vi "plaot slot line.vi"(4 "测试条件out":T3, 6 "粉尘特性":T2, 7 "unit":string, 8 "error in (no error)":errorcluster, 9 "max slop value":cluster{"X":dbl, "Y":dbl}[](array[cluster]), 10 "max slop":dbl, 11 "plot graph":refnum<vi>) -> (0 "error out":errorcluster, 1 "测试条件":string, 2 "intercept":dbl, 3 "dp/dt":string)   [LabVIEW 2011]
panel:
  out "text rect":T1 caption="文本矩形"
  out "rect":T1 caption="矩形"
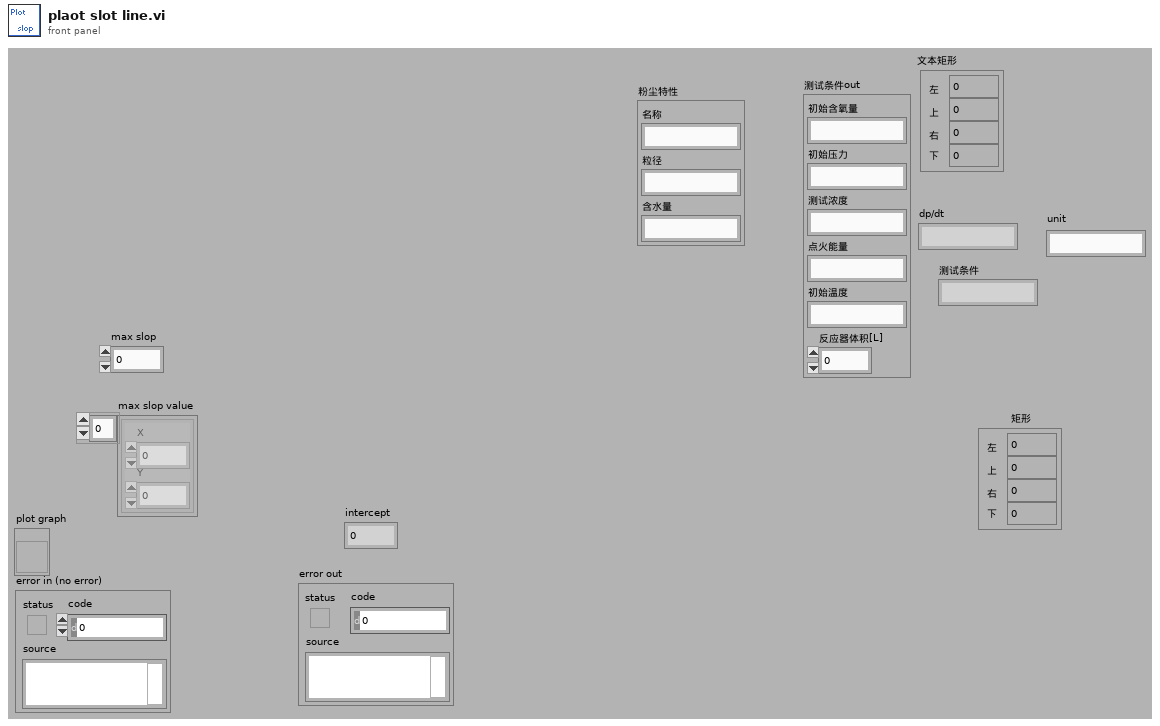
[diagram p1: front panel]
types:
  T1 = cluster{"left":i16, "top":i16, "right":i16, "bottom":i16}
  T2 = typedef "粉尘特性.ctl" = cluster{"名称":string, "粒径":string, "含水量":string}
  T3 = typedef "测试条件.ctl" = cluster{"初始含氧量":string, "初始压力":string, "测试浓度":string, "点火能量":string, "初始温度":string, "反应器体积[L]":dbl}
  T4 = cluster{"horizontal":enum16{"left", "center", "right"}, "vertical":enum16{"top", "center", "bottom"}}
  T5 = enum16{"User-specified Font", "Application Font", "System Font", "Dialog Font"}
  T6 = typedef "LVRectTypeDef.ctl" = cluster{"left":i16, "top":i16, "right":i16, "bottom":i16}
  T7 = typedef "LVPoint32TypeDef.ctl" = cluster{"Horizontal":i32, "Vertical":i32}
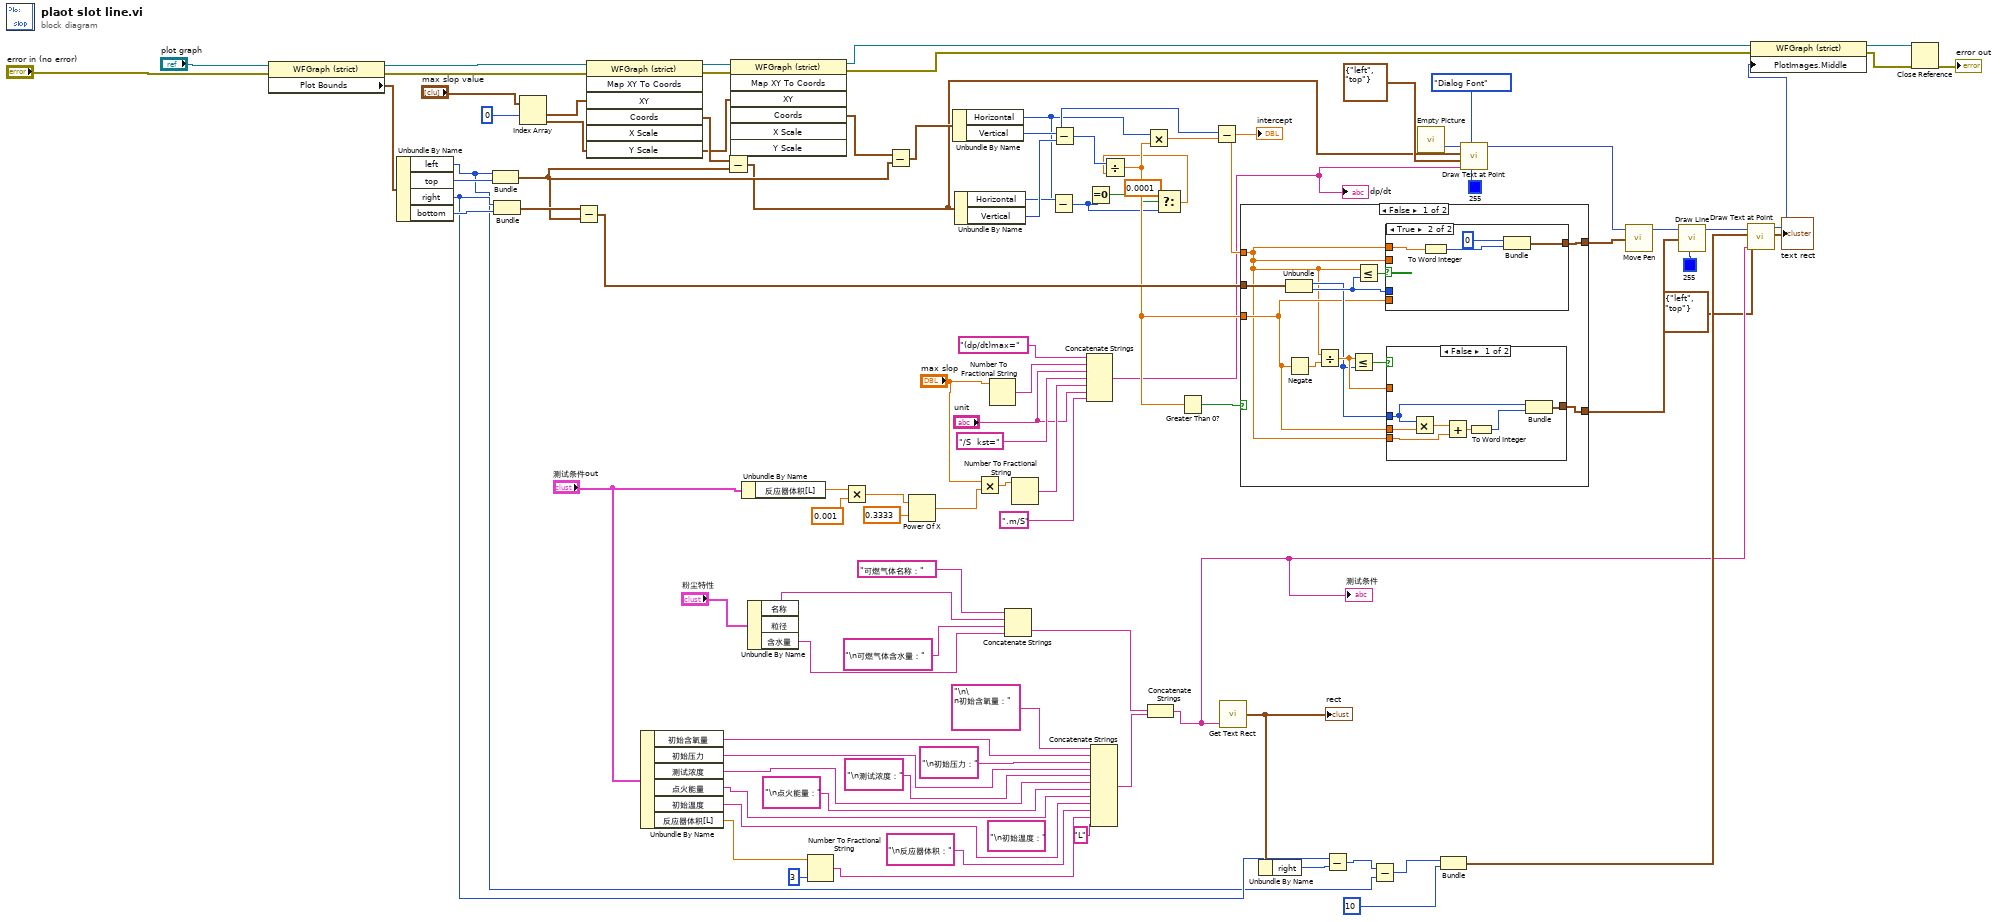
[diagram p0: block diagram]
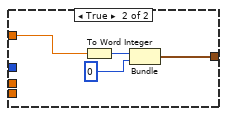
[diagram p2: hidden frame]
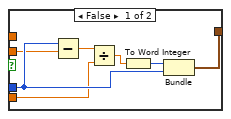
[diagram p3: hidden frame]
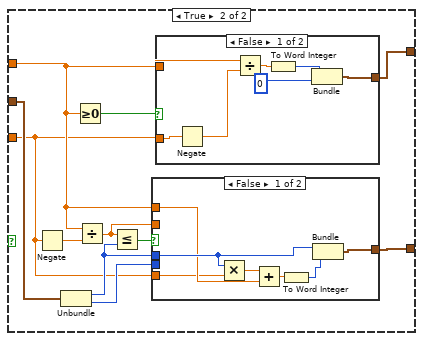
[diagram p4: hidden frame]
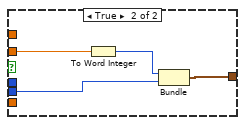
[diagram p5: hidden frame]
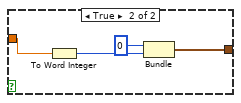
[diagram p6: hidden frame]
diagram:
  (unwired) "\n初始温度：" ("字符串")
  n1 = property class="WFGraph (strict)"(reference="plot graph", error in="error in (no error)") -> (reference out=w89:refnum<vi>, error out=w63:errorcluster, "Plot Bounds"=w88:T6)
  n2 = Unbundle By Name(w88) -> ("left"=w6:i16, "top"=w8:i16, "right"=w10:i16, "bottom"=w83:i16)
  n3 = Bundle("left"=w6, "top"=w8) -> (w81:cluster{"left":i16, "top":i16})  [unwired: 1 out]
  n4 = Bundle("right"=w10, "bottom"=w83) -> (w82:cluster{"right":i16, "bottom":i16})  [unwired: 1 out]
  n5 = Index Array(array="max slop value", index #1=0 ("index")) -> (element #1=w96:cluster{"X":dbl, "Y":dbl}, element #2=w77:cluster{"X":dbl, "Y":dbl})  [unwired: 1 in]
  n6 = Subtract(x=w82, y=w81) -> (x-y=w78:cluster{i16, i16})
  n7 = invoke class="WFGraph (strict)" method="Map XY To Coords"(reference=w89, error in=w63, "XY"=w96) -> (reference out=w92:refnum<vi>, error out=w91:errorcluster, "Coords"=w90:T7)  [unwired: 4 in, 4 out]
  n8 = Unbundle By Name("测试条件out") -> ("初始含氧量"=w30:string, "初始压力"=w27:string, "测试浓度"=w25:string, "点火能量"=w23:string, "初始温度"=w22:string, "反应器体积[L]"=w20:dbl)
  n9 = Subtract(x=w90, y=w81) -> (x-y=w54:T7)
  n10 = invoke class="WFGraph (strict)" method="Map XY To Coords"(reference=w92, error in=w91, "XY"=w77) -> (reference out=w68:refnum<vi>, error out=w62:errorcluster, "Coords"=w87:T7)  [unwired: 4 in, 4 out]
  n11 = Unbundle By Name("测试条件out") -> ("反应器体积[L]"=w40:dbl)
  n12 = Unbundle By Name("粉尘特性") -> ("名称"=w34:string, "含水量"=w31:string)  [unwired: 1 out]
  n13 = Number To Fractional String(number=w20, precision (6)=i16 3 ("精度(6)")) -> (F-format string=w19:string)  [unwired: 2 out]
  n14 = Multiply(x=w40, y=0.001) -> (x*y=w39:dbl)
  n15 = Subtract(x=w87, y=w81) -> (x-y=w71:T7)
  n16 = Power Of X(1:0.3333 ("x"), 2:w39) -> (0:w37:dbl)
  n17 = Unbundle By Name(w71) -> ("Horizontal"=w84:i32, "Vertical"=w86:i32)
  n18 = Unbundle By Name(w54) -> ("Horizontal"=w94:i32, "Vertical"=w95:i32)
  n19 = Multiply(x="max slop", y=w37) -> (x*y=w44:dbl)
  n20 = Number To Fractional String(number="max slop") -> (F-format string=w48:string)  [unwired: 3 out]
  n21 = Concatenate Strings("可燃气体名称：" ("字符串"), w34, "\n可燃气体含水量：" ("字符串"), w31) -> (w18:string)
  n22 = Number To Fractional String(number=w44) -> (F-format string=w45:string)  [unwired: 3 out]
  n23 = Subtract(x=w84, y=w94) -> (x-y=w58:i32)
  n24 = Subtract(x=w86, y=w95) -> (x-y=w93:i32)
  n25 = Concatenate Strings("(dp/dt)max=" ("string"), w48, "unit", "/S  kst=" ("字符串"), w45, "unit", ".m/S" ("字符串")) -> (w69:string)
  "dp/dt" <- w69
  n26 = Equal To 0?(x=w58) -> (x = 0?=w60:bool)
  n27 = Concatenate Strings("\n\n初始含氧量：" ("字符串"), w30, "\n初始压力：" ("字符串"), w27, "\n测试浓度：" ("字符串"), w25, "\n点火能量：" ("字符串"), w23, w22, "\n反应器体积：" ("字符串"), w19, "L" ("字符串")) -> (w17:string)
  n28 = Concatenate Strings(w18, w17) -> (w12:string)
  "测试条件" <- w12
  n29 = Select(t=0.0001, s=w60, f=w58) -> (s? t:f=w57:dbl)
  n30 = Divide(x=w93, y=w57) -> (x/y=w70:dbl)
  n31 = Multiply(x=w84, y=w70) -> (x*y=w85:dbl)
  n32 = Greater Than 0?(x=w70) -> (x > 0?=w80:bool)
  n33 = Subtract(x=w86, y=w85) -> (x-y=w79:dbl)
  "intercept" <- w79
  n34 = call <vilib>:"Get Text Rect.vi"("text"=w12) -> ("rect"=w16:T1)  [unwired: 5 in, 3 out]
  "rect" <- w16
  n35 = case shown="False" w80 {
    tunnel: w79 -> [w99 w131]
    tunnel: w78 -> [w107 w135]
    tunnel: w70 -> [w100 w130]
    tunnel: [w98 w139] -> w74
    tunnel: [w97 w140] -> w76
    frame False {
      n36 = Unbundle(w107) -> (w101:i16, w102:i16)
      n37 = Negate(x=w100) -> (-x=w105:dbl)
      n38 = Divide(x=w99, y=w105) -> (x/y=w103:dbl)
      n39 = Less Or Equal?(x=w103, y=w101) -> (x <= y?=w104:bool)
      n40 = Less Or Equal?(x=w99, y=w102) -> (x <= y?=w106:bool)
      n41 = case shown="True" w106 {
        tunnel: w99 -> [_ w129]
        tunnel: [w125 w126] -> w97
        tunnel: w102 -> [w124 _]
        tunnel: w99 -> [w123 _]
        tunnel: w100 -> [w121 _]
        frame False {
          n42 = Subtract(x=w124, y=w123) -> (x-y=w122:dbl)
          n43 = Divide(x=w122, y=w121) -> (x/y=w120:dbl)
          n44 = To Word Integer(number=w120) -> (16bit integer=w119:i16)
          n45 = Bundle(w119, w124) -> (w125:cluster{i16, i16})  [unwired: 1 out]
        }
        frame True {
          n46 = To Word Integer(number=w129) -> (16bit integer=w127:i16)
          n47 = Bundle(i16 0, w127) -> (w126:cluster{i16, i16})  [unwired: 1 out]
        }
      }
      n48 = case shown="False" w104 {
        tunnel: [w114 w118] -> w98
        tunnel: w103 -> [_ w115]
        tunnel: w101 -> [w113 _]
        tunnel: w100 -> [w112 _]
        tunnel: w99 -> [w110 _]
        frame False {
          n49 = Multiply(x=w113, y=w112) -> (x*y=w111:dbl)
          n50 = Add(x=w111, y=w110) -> (x+y=w109:dbl)
          n51 = To Word Integer(number=w109) -> (16bit integer=w108:i16)
          n52 = Bundle(w113, w108) -> (w114:cluster{i16, i16})  [unwired: 1 out]
        }
        frame True {
          n53 = To Word Integer(number=w115) -> (16bit integer=w116:i16)
          n54 = Bundle(w116, i16 0) -> (w118:cluster{i16, i16})  [unwired: 1 out]
        }
      }
    }
    frame True {
      n55 = Negate(x=w130) -> (-x=w137:dbl)
      n56 = Unbundle(w135) -> (w132:i16, w134:i16)
      n57 = Greater Or Equal To 0?(x=w131) -> (x >= 0?=w138:bool)
      n58 = Divide(x=w131, y=w137) -> (x/y=w133:dbl)
      n59 = Less Or Equal?(x=w133, y=w132) -> (x <= y?=w136:bool)
      n60 = case shown="False" w136 {
        tunnel: [w147 w151] -> w139
        tunnel: w134 -> [_ w150]
        tunnel: w133 -> [_ w149]
        tunnel: w132 -> [w146 _]
        tunnel: w131 -> [w144 _]
        tunnel: w130 -> [w143 _]
        frame False {
          n61 = Multiply(x=w146, y=w143) -> (x*y=w145:dbl)
          n62 = Add(x=w145, y=w144) -> (x+y=w142:dbl)
          n63 = To Word Integer(number=w142) -> (16bit integer=w141:i16)
          n64 = Bundle(w146, w141) -> (w147:cluster{i16, i16})  [unwired: 1 out]
        }
        frame True {
          n65 = To Word Integer(number=w149) -> (16bit integer=w148:i16)
          n66 = Bundle(w148, w150) -> (w151:cluster{i16, i16})  [unwired: 1 out]
        }
      }
      n67 = case shown="False" w138 {
        tunnel: [w158 w162] -> w140
        tunnel: w131 -> [w155 w160]
        tunnel: w130 -> [w154 _]
        frame False {
          n68 = Negate(x=w154) -> (-x=w153:dbl)
          n69 = Divide(x=w155, y=w153) -> (x/y=w152:dbl)
          n70 = To Word Integer(number=w152) -> (16bit integer=w157:i16)
          n71 = Bundle(w157, i16 0) -> (w158:cluster{i16, i16})  [unwired: 1 out]
        }
        frame True {
          n72 = To Word Integer(number=w160) -> (16bit integer=w159:i16)
          n73 = Bundle(i16 0, w159) -> (w162:cluster{i16, i16})  [unwired: 1 out]
        }
      }
    }
  }
  n74 = Unbundle By Name(w16) -> ("right"=w11:i16)
  n75 = Subtract(x=w10, y=w11) -> (x-y=w7:i16)
  n76 = Subtract(x=w7, y=w6) -> (x-y=w3:i16)
  n77 = call "Empty Picture"() -> ("empty picture"=w73:picture)
  n78 = Bundle(w3, "left"=i16 10) -> (w13:cluster{i16, "left":i16})  [unwired: 1 out]
  n79 = call <vilib>:"Draw Text at Point.vi"("text color(black)"=u32 255, "desired font(Application)"=T5."Dialog Font", "text"=w69, "alignment(left, top)"=T4 {"horizontal"=enum."left", "vertical"=enum."top"}, "origin"=w54, "picture"=w73) -> ("new picture"=w53:picture)  [unwired: 3 in, 2 out]
  n80 = call <vilib>:"Move Pen.vi"("new position"=w76, "picture"=w53) -> ("new picture"=w75:picture)  [unwired: 1 in, 2 out]
  n81 = call <vilib>:"Draw Line.vi"("picture"=w75, "end point"=w74, "color(black)"=u32 255) -> ("new picture"=w15:picture)  [unwired: 2 in, 4 out]
  n82 = call <vilib>:"Draw Text at Point.vi"("text"=w12, "alignment(left, top)"=T4 {"horizontal"=enum."left", "vertical"=enum."top"}, "origin"=w13, "picture"=w15) -> ("text rect"=→"text rect":T1, "new picture"=w14:picture)  [unwired: 5 in, 1 out]
  n83 = property class="WFGraph (strict)"(reference=w68, error in=w62, "PlotImages.Middle"=w14) -> (reference out=w67:refnum<vi>, error out=w66:errorcluster)
  n84 = Close Reference(reference=w67, error in (no error)=w66) -> (error out=→"error out":errorcluster)
